vi "IgnoredFailCountDetails_SM.vi"(8 "error in (no error)":errorcluster, 10 "IgnoredCountDetails":cluster{"ReelCount":u64, "TotalCount":u64}, 11 "Inspection Statemachine in":refnum<class "Inspection Statemachine.lvclass">) -> (0 "error out":errorcluster, 3 "Inspection Statemachine out":refnum<class "Inspection Statemachine.lvclass">)   [LabVIEW 2019, in "Inspection Statemachine.lvclass"]
uses:
  Inspection Statemachine.lvclass
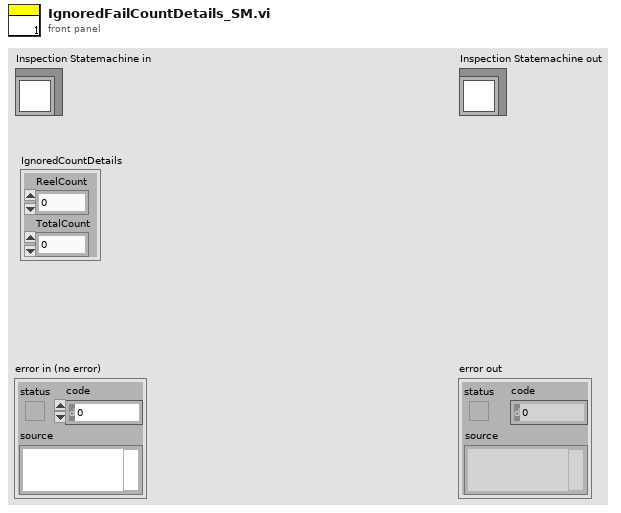
[diagram p1: front panel]
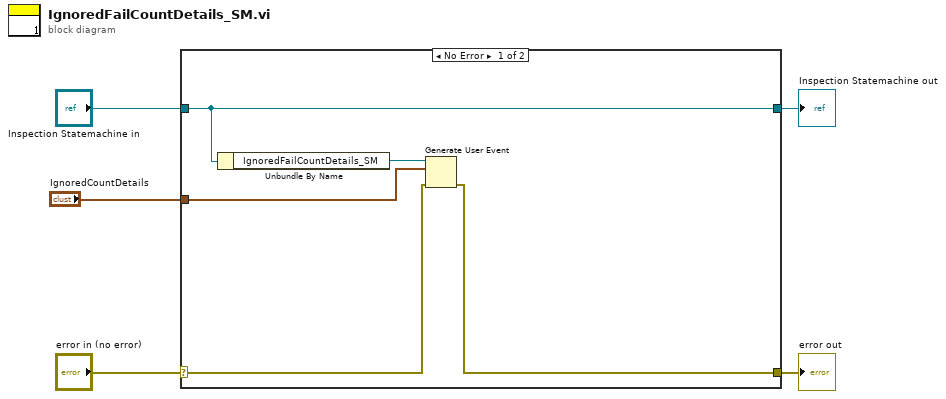
[diagram p0: block diagram]
diagram:
  n1 = case shown="No Error" "error in (no error)" {
    selector: "error in (no error)" -> [w7 w12]
    tunnel: [w6 w12] -> w4
    tunnel: [w10 w11] -> w2
    tunnel: "Inspection Statemachine in" -> [w10 w11]
    tunnel: "IgnoredCountDetails" -> [w8 _]
    frame No Error {
      n2 = Unbundle By Name(w10) -> ("IgnoredFailCountDetails_SM"=w9:refnum<user-event>)
      n3 = Generate User Event(user event=w9, event data cluster=w8, error in=w7) -> (error out=w6:errorcluster)  [unwired: 1 in, 1 out]
    }
    frame Error {
    }
  }
  "error out" <- w4
  "Inspection Statemachine out" <- w2
